vi "Process.vi"(8 "error in":errorcluster, 11 "Logger":refnum<class "Logger.PGSQL.lvclass">) -> (0 "error out":errorcluster, 3 "Logger out":refnum<class "Logger.PGSQL.lvclass">)   [LabVIEW 2019, in "Logger.PGSQL.lvlib" / "Logger.PGSQL.lvclass"]
doc: "---------------------------------------------------------------\nJKI State Machine Objects™\nhttp://jki.net/state-machine-objects/\nCopyright (C) 2005-2015, JKI <info@jki.net>\nALL RIGHTS RESERVED"
uses:
  Logger.PGSQL.lvclass
  <vilib>/JKI/JKI SMO/SMO/SMO.lvclass
  <userlib>/LevyLab/LV-Data/LV-Data.PG/LV-Data.PGSQL.lvclass
  <userlib>/LevyLab/LV-Data/LV-Data.PG/API/Write Variable (one-row).vi
  <userlib>/LevyLab/Logger/Logger/Logger.lvclass
  <userlib>/LevyLab/LV-Data/LV-Data.PG/API/Read Variable (string).vi
  C:/Program Files (x86)/National Instruments/LabVIEW 2019/user.lib/LevyLab/Logger/Logger/Logger.lvclass
  C:/Program Files (x86)/National Instruments/LabVIEW 2019/vi.lib/JKI/JKI SMO/SMO/SMO.lvclass
  <userlib>/LevyLab/Debug/Debug.lvlib
panel:
  out "State History":string
  out "Status":string
  out "Data":variant
  out "Address(es)":string
  # "DB Logger"
  # "For instructions on how to use the JKI State Machine Objects, examples and video tutorials, visit:\nhttp://jki.net/state-machine-objects/\n\nJKI State Machine Objects™\nhttp://jki.net/state-machine-objects/\nCopyright (C) 2005-2015, JKI <info@jki.net>\nALL RIGHTS RESERVED"
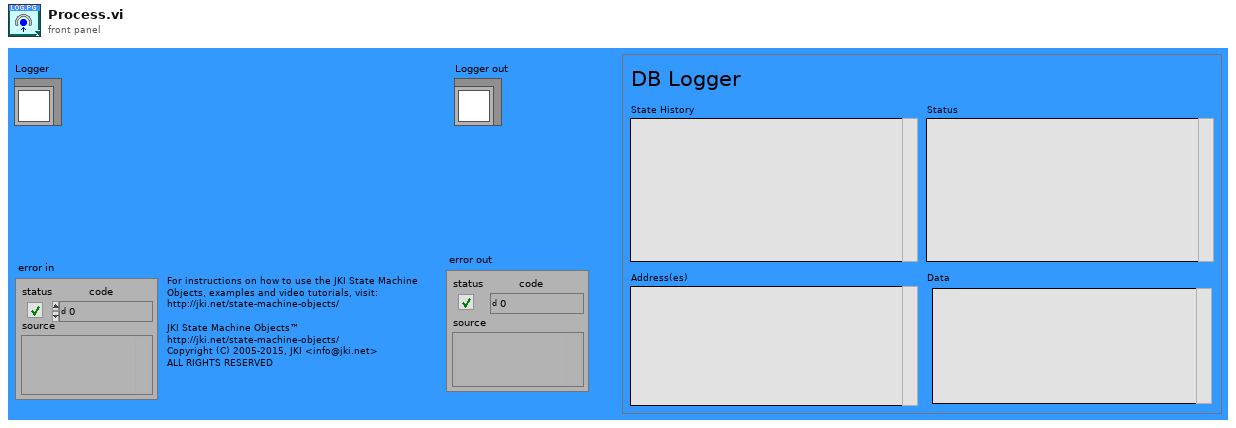
[diagram p1: front panel]
types:
  T1 = enum32{"invalid app kind", "Development System", "Run Time System", "Student Edition", "Embedded LabVIEW", "Evaluation", "Custom"}
  T2 = enum32{"Invalid", "Standard", "Closed", "Hidden", "Minimized", "Maximized"}
  T3 = cluster{"Core":cluster{"Current VI Reference":refnum<vi>, "Close Panel on Exit?":bool, "Last Error":cluster{"error":errorcluster, "previous state":string, "remaining states":string}, "Shutdown?":bool}, "SelfRef":refnum<class "Logger.PGSQL.lvclass">, "Data.PGSQL":refnum<class "LV-Data.PGSQL.lvclass">, "variable address":string, "data in":variant, "data out":variant, "Time":timestamp, "UI Behavior":string, "wait":u32}
  T4 = cluster{"Current VI Reference":refnum<vi>, "Close Panel on Exit?":bool, "Last Error":cluster{"error":errorcluster, "previous state":string, "remaining states":string}, "Shutdown?":bool}
  T5 = typedef "Debug.lvlib/Attribute.Debug.lvclass/DebugBehavior.ctl" = enum16{"Normal", "Debug"}
  T6 = typedef "smo.lvlib/SMO.lvclass/Protected Events.ctl" = cluster{"StopProcesses":refnum<user-event>, "AbortProcesses":refnum<user-event>, "Config Changed":refnum<user-event>, "Dependency":refnum<user-event>}
  T7 = typedef "Logger.PGSQL.lvlib/Logger.PGSQL.lvclass/PrivateEvents--Cluster.ctl" = cluster{"Set Address":refnum<user-event>, "Write Variable":refnum<user-event>, "Read Variable":refnum<user-event>}
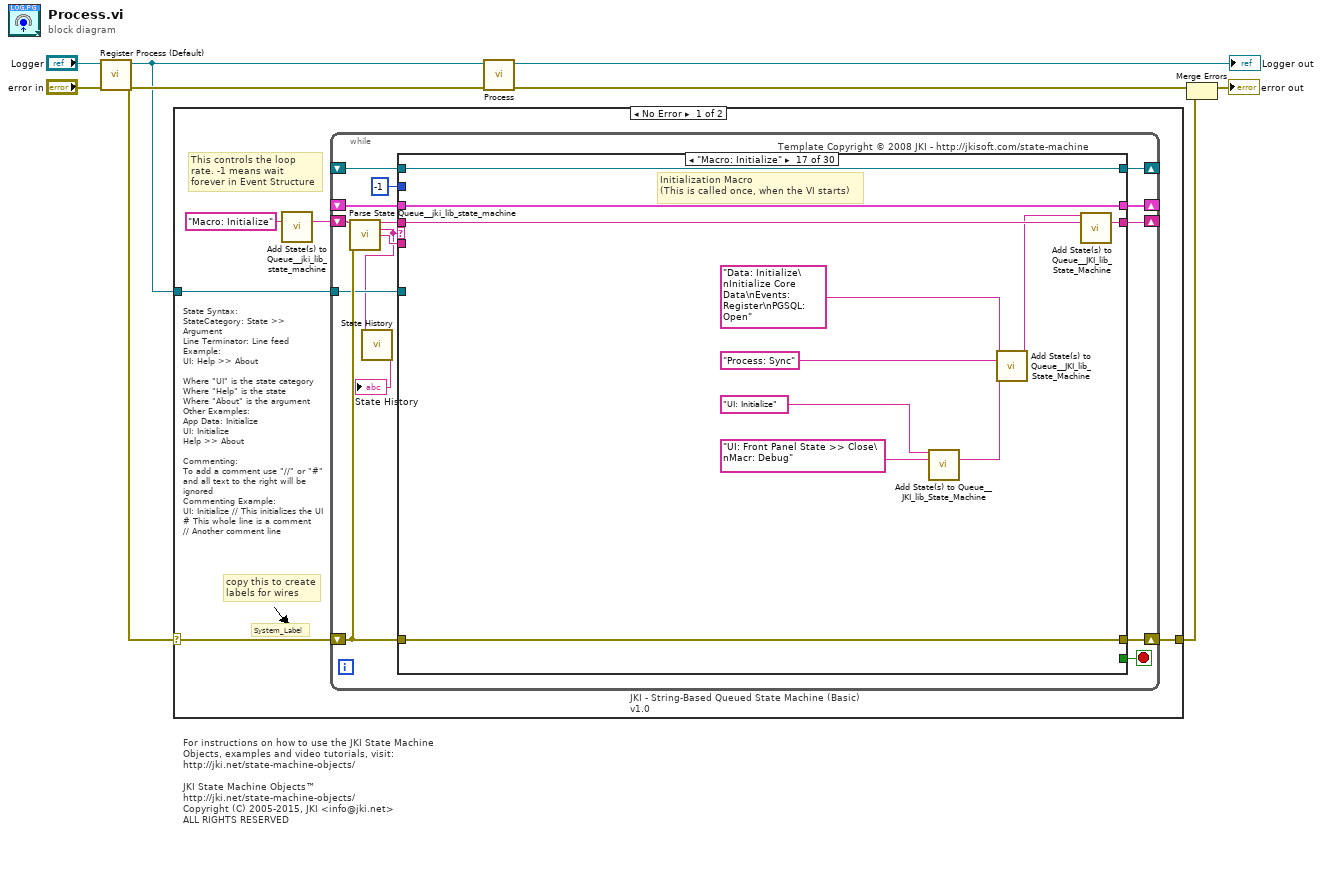
[diagram p0: block diagram]
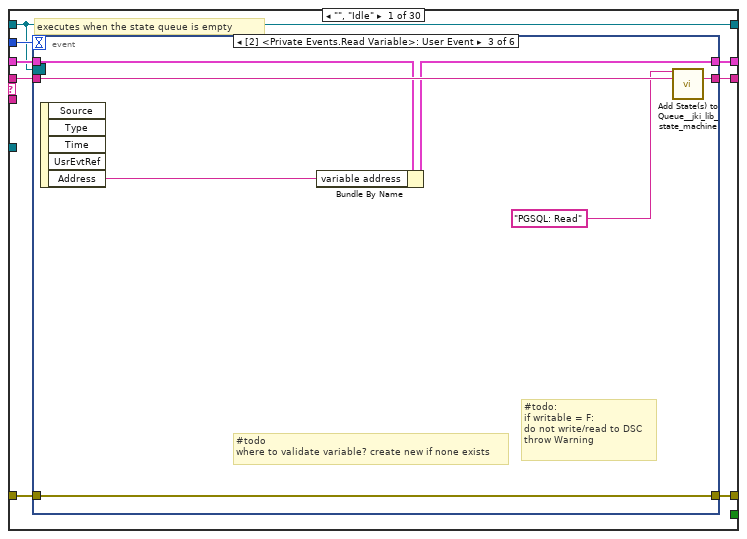
[diagram p2: hidden frame]
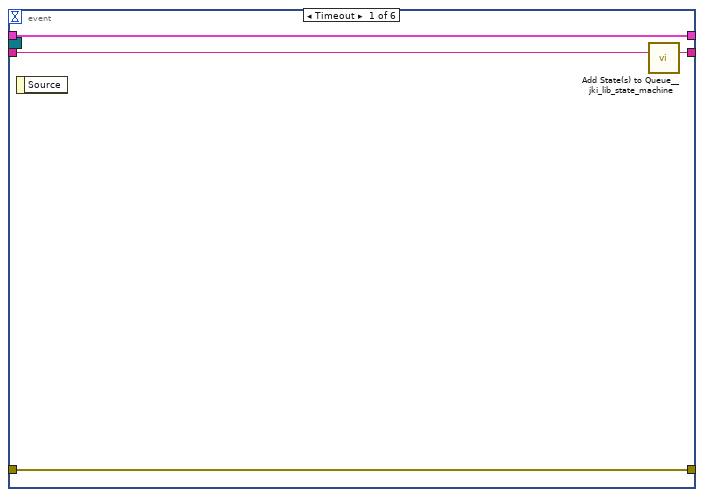
[diagram p3: hidden frame]
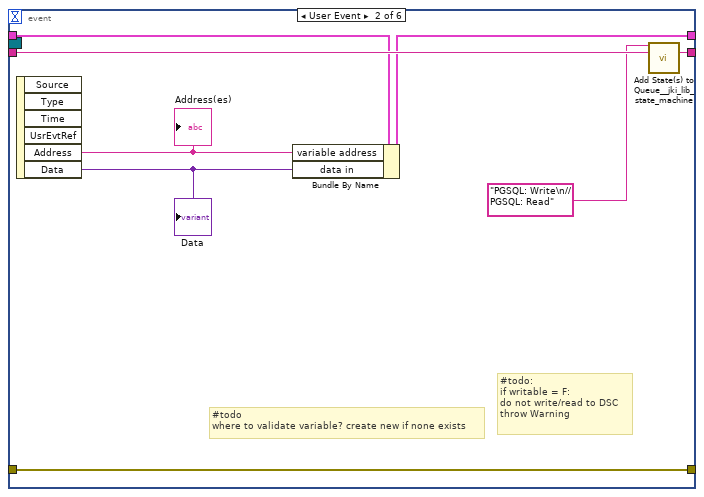
[diagram p4: hidden frame]
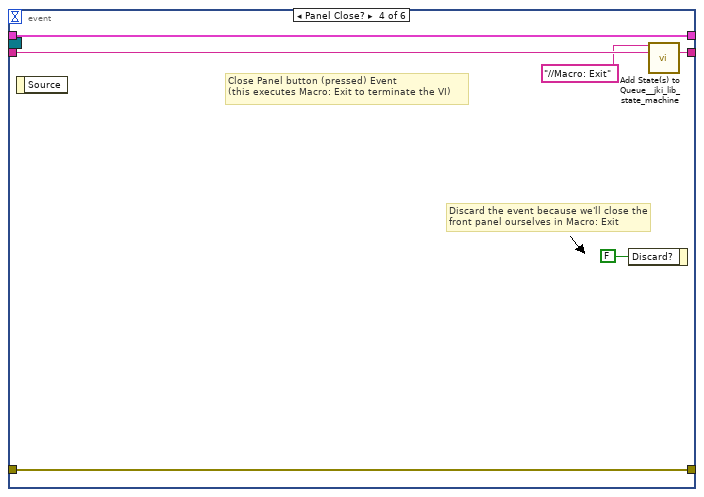
[diagram p5: hidden frame]
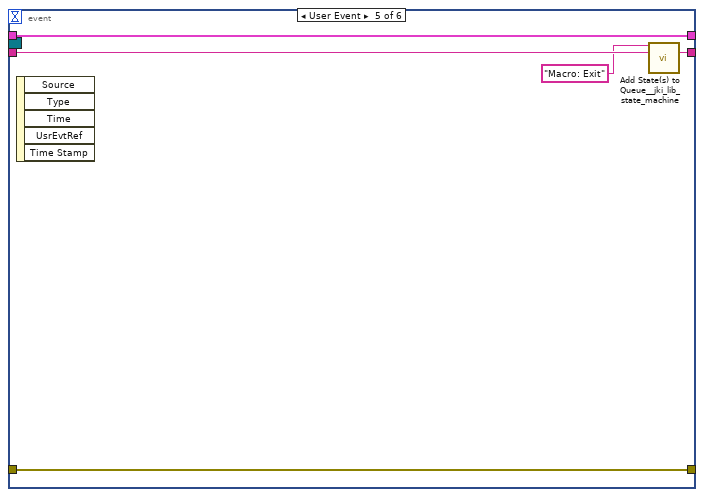
[diagram p6: hidden frame]
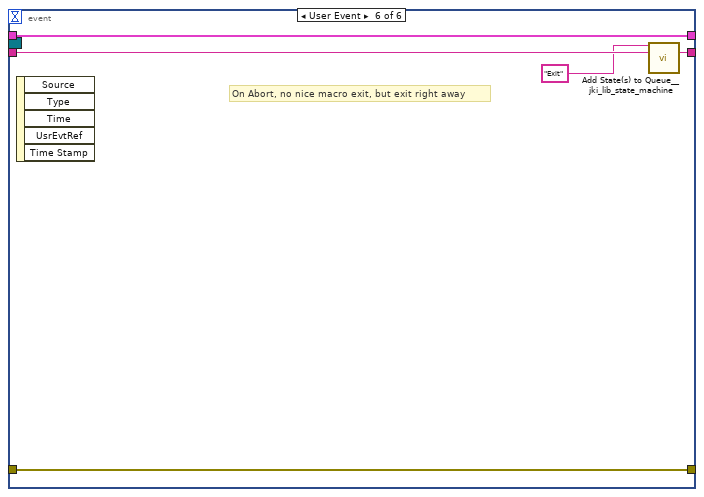
[diagram p7: hidden frame]
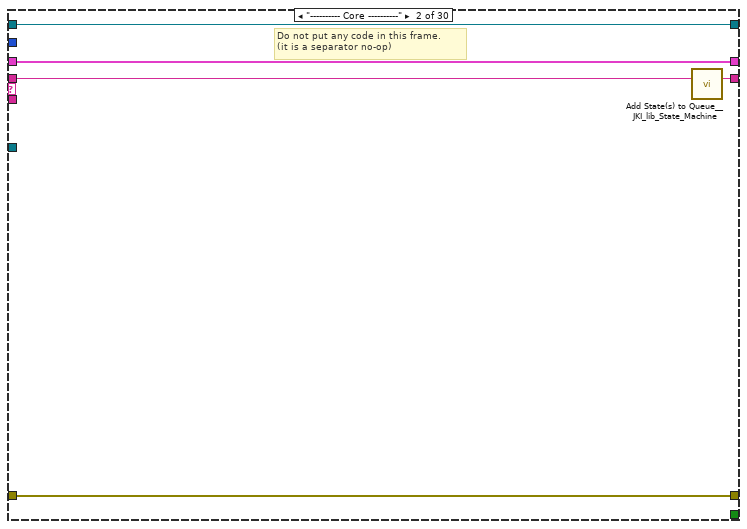
[diagram p8: hidden frame]
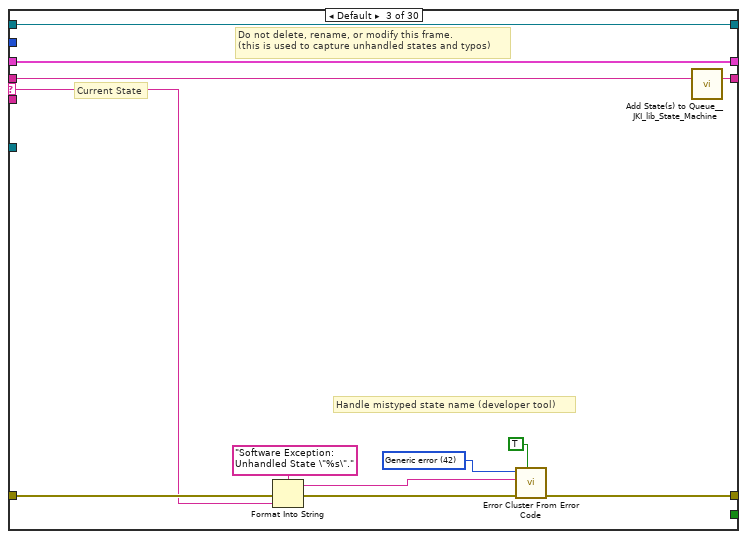
[diagram p9: hidden frame]
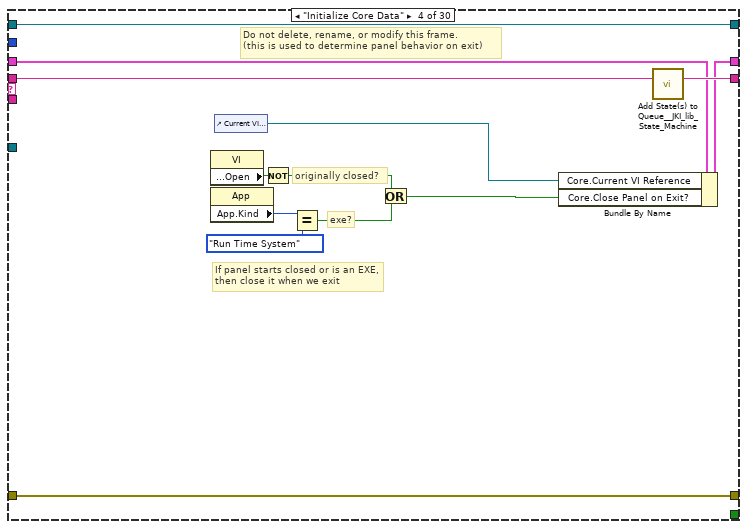
[diagram p10: hidden frame]
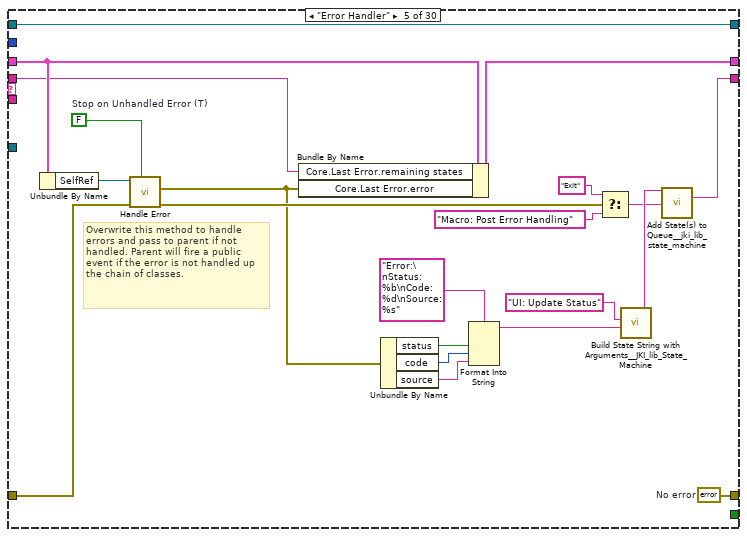
[diagram p11: hidden frame]
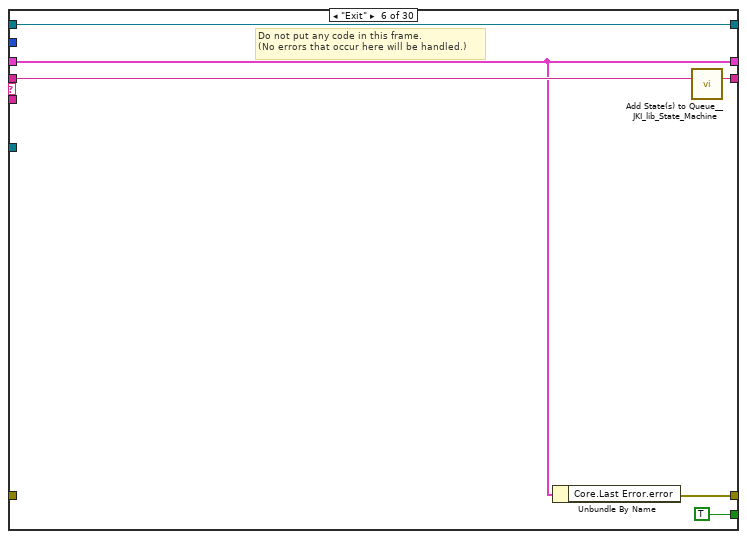
[diagram p12: hidden frame]
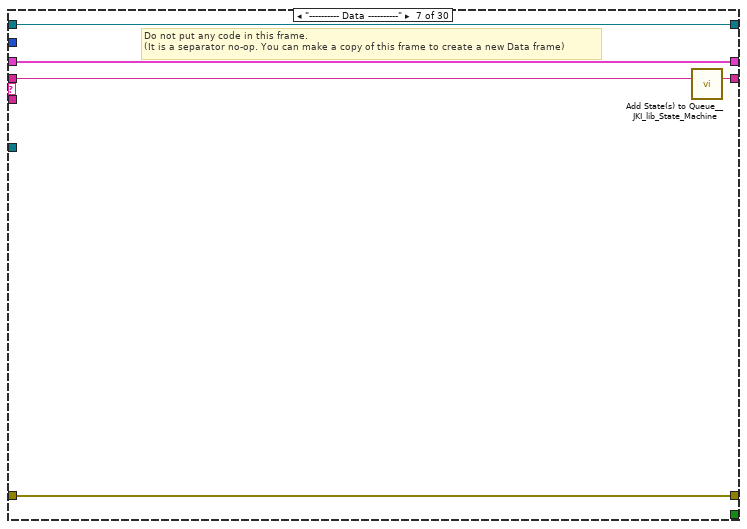
[diagram p13: hidden frame]
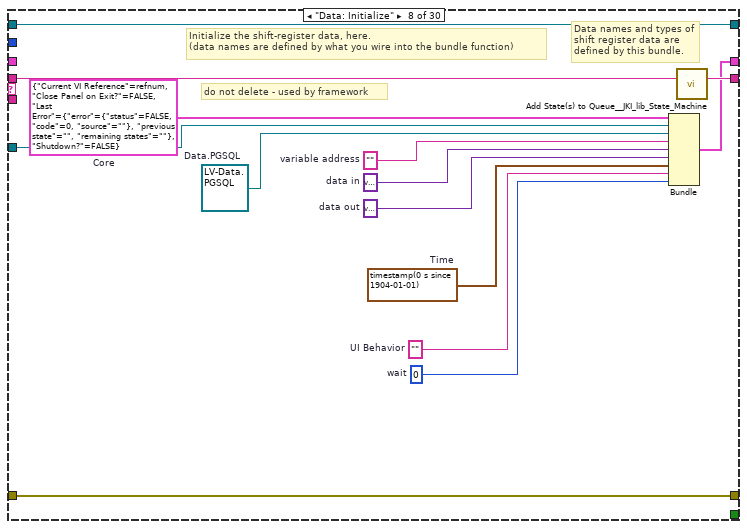
[diagram p14: hidden frame]
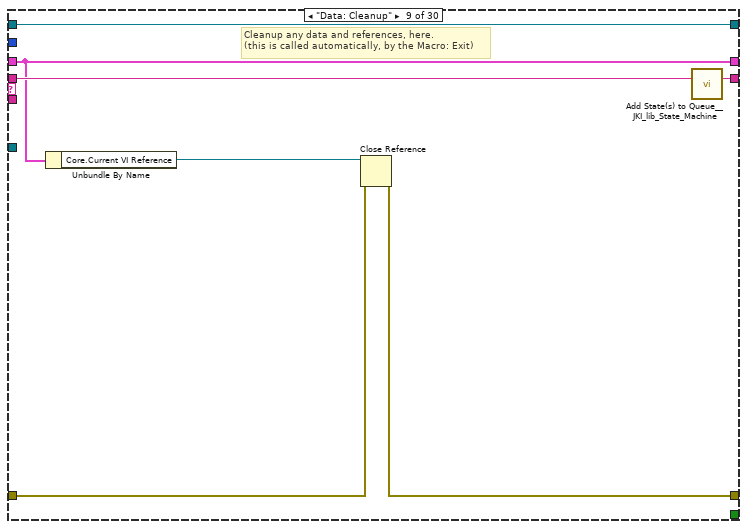
[diagram p15: hidden frame]
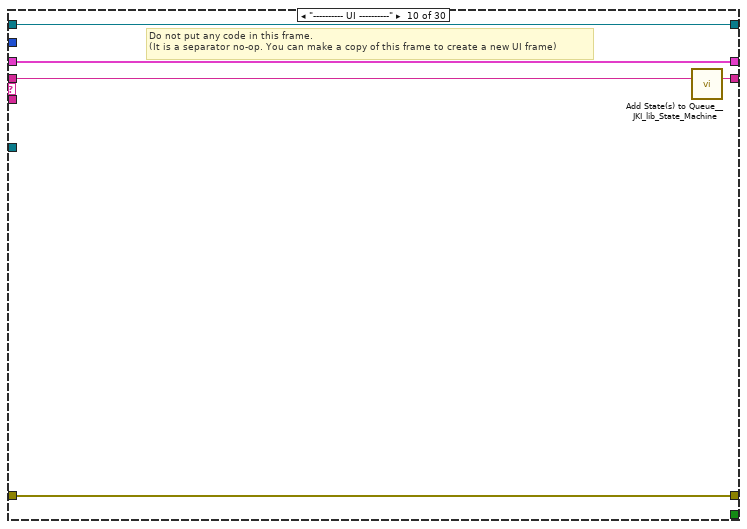
[diagram p16: hidden frame]
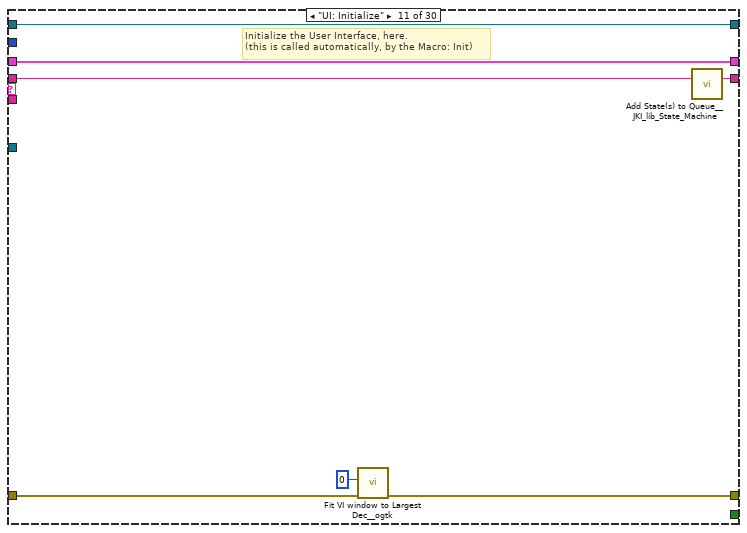
[diagram p17: hidden frame]
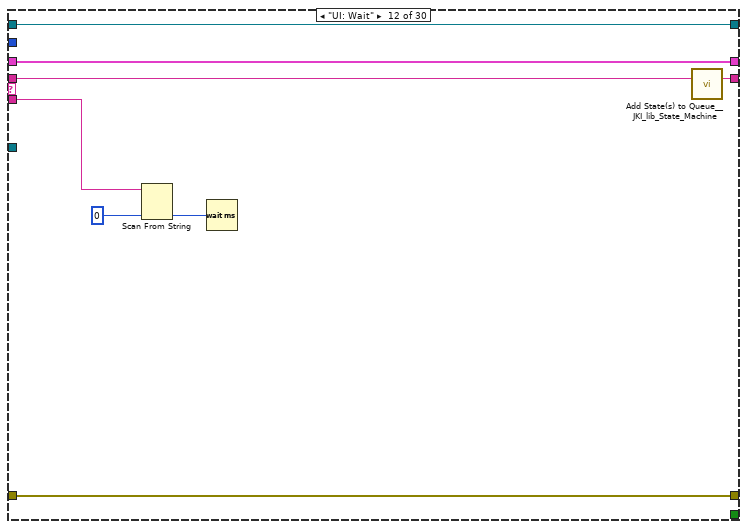
[diagram p18: hidden frame]
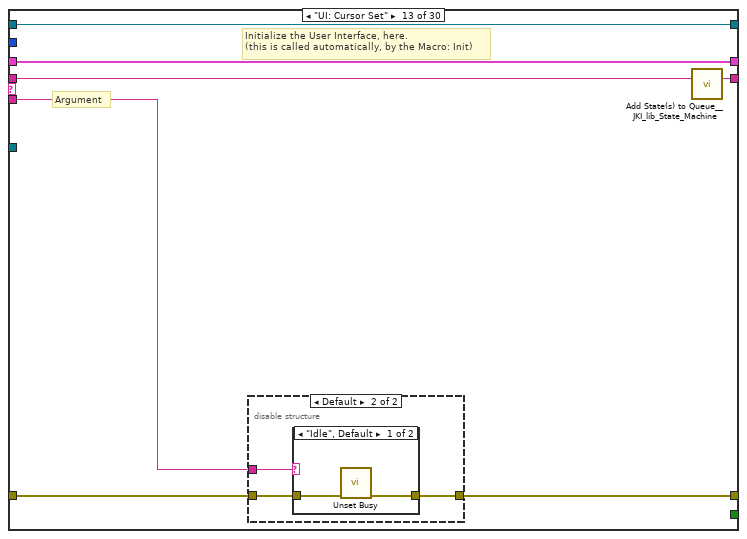
[diagram p19: hidden frame]
diagram:
  # "For instructions on how to use the JKI State Machine Objects, examples and video tutorials, visit:\nhttp://jki.net/state-machine-objects/\n\nJKI State Machine Objects™\nhttp://jki.net/state-machine-objects/\nCopyright (C) 2005-2015, JKI <info@jki.net>\nALL RIGHTS RESERVED"
  n1 = call <vilib>:"Register Process (Default).vi"("error in (no error)"="error in", "SMO"="Logger") -> ("error out"=w5:errorcluster, "SelfRef"=w4:refnum<class "Logger.PGSQL.lvclass">)  [unwired: 8 in]
  n2 = case shown="No Error" w5 {
    selector: w5 -> [w10 w424]
    tunnel: w4 -> [w11 _]
    tunnel: [w9 w424] -> w2
    frame No Error {
      # "State Syntax:\nStateCategory: State >> Argument\nLine Terminator: Line feed\nExample:\nUI: Help >> About\n\nWhere \"UI\" is the state category\nWhere \"Help\" is the state\nWhere \"About\" is the argument\nOther Examples:\nApp Data: Initialize\nUI: Initialize\nHelp >> About\n\nCommenting:\nTo add a comment use \"//\" or \"#\" and all text to the right will be ignored\nCommenting Example:\nUI: Initialize // This initializes the UI\n# This whole line is a comment\n// Another comment line"
      # "copy this to create labels for wires"
      # "This controls the loop rate. -1 means wait forever in Event Structure"
      # "System_Label"
      n3 = call <vilib>:"Add State(s) to Queue__jki_lib_state_machine.vi"("State(s) in (\"\")"="Macro: Initialize") -> ("States Out"=w13:string)  [unwired: 14 in]
      n4 = while "JKI - String-Based Queued State Machine (Basic) v1.0" {
        shift-right: [w22] -> _
        shift-left: _ -> [w21]
        shift-right: [w25] -> w9
        shift-left: w10 -> [w19]
        shift-right: [w24] -> _
        shift-left: w13 -> [w26]
        tunnel: w11 -> [w18]
        shift-right: [w17] -> _
        shift-left: _ -> [w16]
        stop <- w23 stop-if-true
        # "Template Copyright © 2008 JKI - http://jkisoft.com/state-machine"
        n5 = call <vilib>:"Parse State Queue__jki_lib_state_machine.vi"("State Queue"=w26, "Error In (no error)"=w19) -> ("Remaining States"=w28:string, "Current State"=w14:string, "Arguments"=w27:string)  [unwired: 11 in]
        n6 = call <userlib>:"State History.vi"("Current State"=w14) -> ("History"=→"State History":string)  [unwired: 10 in]
        n7 = case shown="\"Macro: Initialize\"" w14 {
          selector: w14 -> [_ _ w78 _ _ _ _ _ _ _ _ _ _ _ _ _ _ _ _ _ _ _ _ _ _ _ _ _ _ _]
          tunnel: w28 -> [w36 w76 w82 w101 w108 w128 w133 w147 w154 w159 w166 w174 w181 w196 w204 w236 w247 w261 w278 w298 w303 w314 w319 w332 w338 w343 w352 w376 w406 w423]
          tunnel: w27 -> [_ _ _ _ _ _ _ _ _ _ _ w168 w175 w190 w198 _ _ _ _ _ _ _ _ _ _ _ _ _ _ _]
          tunnel: w21 -> [w34 w73 w80 w92 w118 w124 w130 _ w149 w156 w164 w171 w179 w193 w200 w233 w241 w249 w268 w283 w300 w311 w316 w330 w336 w341 w344 w371 w399 w418]
          tunnel: [w33 w74 w84 w98 w119 w123 w131 w136 w150 w157 w162 w172 w176 w194 w201 w234 w237 w259 w276 w296 w301 w305 w317 w325 w334 w339 w347 w373 w403 w415] -> w25
          tunnel: w19 -> [w32 w74 w83 w98 w120 _ w131 w136 w151 w157 w161 w172 w177 w194 w202 w234 w237 w259 w276 w296 w301 w306 w317 w326 w334 w339 w345 w368 w400 w416]
          tunnel: [w35 w75 w81 w100 w104 w127 w132 w146 w153 w158 w165 w173 w180 w195 w203 w235 w246 w260 w277 w297 w302 w313 w318 w331 w337 w342 w351 w375 w405 w422] -> w24
          tunnel: [_ _ _ _ _ TRUE _ _ _ _ _ _ _ _ _ _ _ _ _ _ _ _ _ _ _ _ _ _ _ _] -> w23
          tunnel: [w31 w73 w80 w99 w117 w124 w130 w145 w149 w156 w164 w171 w179 w193 w200 w233 w241 w250 w269 w284 w300 w311 w316 w330 w336 w341 w349 w370 w399 w417] -> w22
          tunnel: -1 ("Timeout") -> [w30 _ _ _ _ _ _ _ _ _ _ _ _ _ _ _ _ _ _ _ _ _ _ _ _ _ _ _ _ _]
          tunnel: w18 -> [_ _ _ _ _ _ _ w137 _ _ _ _ _ _ _ _ _ _ _ _ _ _ _ _ _ _ _ _ _ _]
          tunnel: [w29 w72 w77 w89 w122 w125 w129 w144 w148 w155 w163 w170 w178 w192 w197 w232 w245 w258 w275 w291 w299 w312 w315 w329 w335 w340 w350 w374 w404 w421] -> w17
          tunnel: w16 -> [w29 w72 w77 w89 w122 w125 w129 w144 w148 w155 w163 w170 w178 w192 w197 w232 w245 w258 w275 w291 w299 w312 w315 _ w335 w340 w350 w374 w404 w421]
          frame "", "Idle" {
            # "executes when the state queue is empty"
            n8 = event shown="[2] <Private Events.Read Variable>: User Event" {
              selector: w29 -> [_ _ _ _ _ _]
              dyn-events: _ -> [_ _ _ _ _ _]
              timeout: w30 -> [_ _ _ _ _ _]
              tunnel: w36 -> [w40 w48 w55 w61 w66 w71]
              tunnel: [w39 w47 w54 w60 w65 w70] -> w35
              tunnel: w34 -> [w38 w45 w52 w58 w63 w68]
              tunnel: [w37 w46 w53 w59 w64 w69] -> w33
              tunnel: w32 -> [w37 w46 w53 w59 w64 w69]
              tunnel: [w38 w44 w51 w58 w63 w68] -> w31
              event Timeout {
                n9 = event-data() -> ()  [unwired: 1 in, 1 out]
                n10 = call <vilib>:"Add State(s) to Queue__jki_lib_state_machine.vi"("State(s) in (\"\")"=w40) -> ("States Out"=w39:string)  [unwired: 14 in]
              }
              event User Event {
                # "#todo:\nif writable = F:\ndo not write/read to DSC\nthrow Warning"
                # "#todo\nwhere to validate variable? create new if none exists"
                n11 = event-data() -> ("Address"=w41:string, "Data"=w42:variant)  [unwired: 1 in, 4 out]
                "Address(es)" <- w41
                "Data" <- w42
                n12 = Bundle By Name(cluster=w45, "variable address"=w41, "data in"=w42) -> (w44:T3)
                n13 = call <vilib>:"Add State(s) to Queue__jki_lib_state_machine.vi"("State(s) in Front (\"\")"="PGSQL: Write\n//PGSQL: Read" ("State(s) in Front (\"\")"), "State(s) in (\"\")"=w48) -> ("States Out"=w47:string)  [unwired: 13 in]
              }
              event User Event {
                # "#todo:\nif writable = F:\ndo not write/read to DSC\nthrow Warning"
                # "#todo\nwhere to validate variable? create new if none exists"
                n14 = event-data() -> ("Address"=w49:string)  [unwired: 1 in, 4 out]
                n15 = Bundle By Name(cluster=w52, "variable address"=w49) -> (w51:T3)
                n16 = call <vilib>:"Add State(s) to Queue__jki_lib_state_machine.vi"("State(s) in Front (\"\")"="PGSQL: Read" ("State(s) in Front (\"\")"), "State(s) in (\"\")"=w55) -> ("States Out"=w54:string)  [unwired: 13 in]
              }
              event Panel Close? {
                # "Discard the event because we'll close the front panel ourselves in Macro: Exit"
                # "Close Panel button (pressed) Event\n(this executes Macro: Exit to terminate the VI)"
                n17 = event-data() -> ()  [unwired: 1 in, 1 out]
                n18 = event-data("Discard?"=FALSE) -> ()  [unwired: 1 in, 1 out]
                n19 = call <vilib>:"Add State(s) to Queue__jki_lib_state_machine.vi"("State(s) in Front (\"\")"="//Macro: Exit", "State(s) in (\"\")"=w61) -> ("States Out"=w60:string)  [unwired: 13 in]
              }
              event User Event {
                n20 = event-data() -> ()  [unwired: 1 in, 5 out]
                n21 = call <vilib>:"Add State(s) to Queue__jki_lib_state_machine.vi"("State(s) in Front (\"\")"="Macro: Exit", "State(s) in (\"\")"=w66) -> ("States Out"=w65:string)  [unwired: 13 in]
              }
              event User Event {
                # "On Abort, no nice macro exit, but exit right away"
                n22 = event-data() -> ()  [unwired: 1 in, 5 out]
                n23 = call <vilib>:"Add State(s) to Queue__jki_lib_state_machine.vi"("State(s) in Front (\"\")"="Exit", "State(s) in (\"\")"=w71) -> ("States Out"=w70:string)  [unwired: 13 in]
              }
            }
          }
          frame "---------- Core ----------" {
            # "Do not put any code in this frame.\n(it is a separator no-op)"
            n24 = call <vilib>:"Add State(s) to Queue__JKI_lib_State_Machine.vi"("State(s) in (\"\")"=w76) -> ("States Out"=w75:string)  [unwired: 14 in]
          }
          frame Default {
            w87 = 42 items=["No error", "Argument error", "Memory is full", "Out of zone", "End of file", "File already open", "Generic file I/O error", "File not found", "File permission error", "Disk is full", "Duplicate path", "Too many files open", "System feature not enabled", "Resource file not found", "Cannot add resource", "Resource not found", "Image not found", "Image memory error", "Pen does not exist", "Config type invalid", "Config token not found", "Config parse error", "Config memory error", "Bad external code format", "Bad external code offset", "External code not present", "Null window", "Destroy window error", "Null menu", "Print aborted", "Bad print record", "Print driver error", "Windows error during printing", "Memory error during printing", "Print dialog error", "Generic print error", "Invalid device refnum", "Device not found", "Device parameter error", "Device unit error", "Cannot open device", "Device call aborted", "Generic error", "Cancelled by user", "Object ID too low", "Object ID too high", "Object not in heap", "Unknown heap", "Unknown object (invalid DefProc)", "Unknown object (DefProc not in table)", "Message out of range", "Invalid (null) method", "Unknown message", "Manager call not supported", "Bad address", "Network operation in progress", "Network operation timed out", "Connection is busy", "Network attribute not supported", "Network error", "Address in use", "System out of memory", "Connection aborted", "Connection refused", "Not connected", "Already connected", "Connection closed", "Initialization error (interapplication manager)", "Bad occurrence", "Wait on unbound occurrence handler", "Occurrence queue overflow", "Datalog type conflict", "Unused", "Unrecognized type (interapplication manager)", "Memory corrupt", "Failed to make temporary DLL", "Old CIN version", "Drag socket not found", "Failed to load drop-object", "Failed to register OLE object", "Failed to release OLE object", "Format specifier type mismatch", "Unknown format specifier", "Too few format specifiers", "Too many format specifiers", "Scan failed", "Newer CIN version", "Error converting to variant", "Runtime menu error", "Password tampered", "Variant attribute not found", "Incompatible variant data type", "Event data is not available", "Event Store is not present", "Occurrence is not found", "Event Queue is not created", "Event info is not available", "Refnum passed is NULL", "Error retrieving Class GUID", "Error retrieving CoClass GUID", "Error retrieving TypeLib GUID.", "Bad built application magic bytes.", "Specific driver is different from the specific driver associated with the Logical Name.", "There is no session opened to the class driver.", "Max Error", "MAX - Error with config objects", "MAX - Error loading configuration", "MAX - Group not supported"]
            # "Current State"
            # "Do not delete, rename, or modify this frame.\n(this is used to capture unhandled states and typos)"
            # "Handle mistyped state name (developer tool)"
            n25 = Format Into String(format string="Software Exception: Unhandled State \"%s\"." ("message"), error in=w83, w78) -> (resulting string=w86:string, error out=w85:errorcluster)  [unwired: 1 in]
            n26 = call <vilib>:"Error Cluster From Error Code.vi"("show call chain? (False)"=TRUE, "error in (no error)"=w85, "error message (\"\")"=w86, "error code (0)"=w87) -> ("error out"=w84:errorcluster)  [unwired: 5 in]
            n27 = call <vilib>:"Add State(s) to Queue__JKI_lib_State_Machine.vi"("State(s) in (\"\")"=w82) -> ("States Out"=w81:string)  [unwired: 14 in]
          }
          frame "Initialize Core Data" {
            # "Do not delete, rename, or modify this frame.\n(this is used to determine panel behavior on exit)"
            # "originally closed?"
            # "exe?"
            # "If panel starts closed or is an EXE, then close it when we exit"
            n28 = property class="VI"() -> ("Front Panel.Open"=w97:bool)  [unwired: 2 in, 2 out]
            n29 = property class="App"() -> ("App.Kind"=w96:T1)  [unwired: 2 in, 2 out]
            n30 = control-ref of="Current VI Reference"() -> (w90:refnum<vi>)
            n31 = Not(x=w97) -> (.not. x?=w94:bool)
            n32 = Equal?(x=w96, y=T1."Run Time System" ("Application:Kind")) -> (x = y?=w93:bool)
            n33 = Or(x=w94, y=w93) -> (x .or. y?=w91:bool)
            n34 = Bundle By Name(cluster=w92, "Core.Current VI Reference"=w90, "Core.Close Panel on Exit?"=w91) -> (w99:T3)
            n35 = call <vilib>:"Add State(s) to Queue__JKI_lib_State_Machine.vi"("State(s) in (\"\")"=w101) -> ("States Out"=w100:string)  [unwired: 14 in]
          }
          frame "Error Handler" {
            w114 = FALSE  # Stop on Unhandled Error (T)
            w119 = errorcluster {"status"=FALSE, "code"=0, "source"=""}  # No error
            # "Overwrite this method to handle errors and pass to parent if not handled. Parent will fire a public event if the error is not handled up the chain of classes."
            n36 = Unbundle By Name(w118) -> ("SelfRef"=w121:refnum<class "Logger.PGSQL.lvclass">)
            n37 = call-dynamic "Handle Error.vi"("Stop on Unhandled Error (T)"=w114, "error in"=w120, "SMO"=w121) -> ("handling error"=w115:errorcluster, "Unhandled error"=w113:errorcluster)  [unwired: 6 in, 1 out]
            n38 = Bundle By Name(cluster=w118, "Core.Last Error.remaining states"=w108, "Core.Last Error.error"=w113) -> (w117:T3)
            n39 = Unbundle By Name(w113) -> ("status"=w112:bool, "code"=w110:i32, "source"=w109:string)
            n40 = Format Into String(format string="Error:\nStatus: %b\nCode: %d\nSource: %s", w112, w110, w109) -> (resulting string=w103:string)  [unwired: 2 in, 1 out]
            n41 = Select(t="Exit", s=w115, f="Macro: Post Error Handling") -> (s? t:f=w105:string)
            n42 = call <vilib>:"Build State String with Arguments__JKI_lib_State_Machine.vi"("Arguments (\"\")"=w103, "State"="UI: Update Status") -> ("State with Arguments"=w106:string)  [unwired: 4 in]
            n43 = call <vilib>:"Add State(s) to Queue__jki_lib_state_machine.vi"("State(s) in Front (\"\")"=w106, "State(s) at Back (\"\")"=w105) -> ("States Out"=w104:string)  [unwired: 13 in]
          }
          frame "Exit" {
            # "Do not put any code in this frame.\n(No errors that occur here will be handled.)"
            n44 = Unbundle By Name(w124) -> ("Core.Last Error.error"=w123:errorcluster)
            n45 = call <vilib>:"Add State(s) to Queue__JKI_lib_State_Machine.vi"("State(s) in (\"\")"=w128) -> ("States Out"=w127:string)  [unwired: 14 in]
          }
          frame "---------- Data ----------" {
            # "Do not put any code in this frame.\n(It is a separator no-op. You can make a copy of this frame to create a new Data frame)"
            n46 = call <vilib>:"Add State(s) to Queue__JKI_lib_State_Machine.vi"("State(s) in (\"\")"=w133) -> ("States Out"=w132:string)  [unwired: 14 in]
          }
          frame "Data: Initialize" {
            w134 = u32 0  # wait
            w135 = ""  # UI Behavior
            w138 = timestamp(0 s since 1904-01-01)  # Time
            w139 = refnum<class "LV-Data.PGSQL.lvclass"> refnum  # Data.PGSQL
            w140 = variant  # data out
            w141 = variant  # data in
            w142 = ""  # variable address
            w143 = T4 {"Current VI Reference"=refnum, "Close Panel on Exit?"=FALSE, "Last Error"={"error"={"status"=FALSE, "code"=0, "source"=""}, "previous state"="", "remaining states"=""}, "Shutdown?"=FALSE}  # Core
            # "do not delete - used by framework"
            # "Data names and types of shift register data are defined by this bundle."
            # "Initialize the shift-register data, here.\n(data names are defined by what you wire into the bundle function)"
            n47 = Bundle("Core"=w143, "SelfRef"=w137, "Data.PGSQL"=w139, "variable address"=w142, "data in"=w141, "data out"=w140, "Time"=w138, "UI Behavior"=w135, "wait"=w134) -> (w145:T3)  [unwired: 1 in]
            n48 = call <vilib>:"Add State(s) to Queue__JKI_lib_State_Machine.vi"("State(s) in (\"\")"=w147) -> ("States Out"=w146:string)  [unwired: 14 in]
          }
          frame "Data: Cleanup" {
            # "Cleanup any data and references, here.\n(this is called automatically, by the Macro: Exit)"
            n49 = Unbundle By Name(w149) -> ("Core.Current VI Reference"=w152:refnum<vi>)
            n50 = Close Reference(reference=w152, error in (no error)=w151) -> (error out=w150:errorcluster)
            n51 = call <vilib>:"Add State(s) to Queue__JKI_lib_State_Machine.vi"("State(s) in (\"\")"=w154) -> ("States Out"=w153:string)  [unwired: 14 in]
          }
          frame "---------- UI ----------" {
            # "Do not put any code in this frame.\n(It is a separator no-op. You can make a copy of this frame to create a new UI frame)"
            n52 = call <vilib>:"Add State(s) to Queue__JKI_lib_State_Machine.vi"("State(s) in (\"\")"=w159) -> ("States Out"=w158:string)  [unwired: 14 in]
          }
          frame "UI: Initialize" {
            # "Initialize the User Interface, here.\n(this is called automatically, by the Macro: Init)"
            n53 = call <userlib>:"Fit VI window to Largest Dec__ogtk.vi"("error in (no error)"=w161, "border spacing (2 px)"=0) -> ("error out"=w162:errorcluster)  [unwired: 4 in, 1 out]
            n54 = call <vilib>:"Add State(s) to Queue__JKI_lib_State_Machine.vi"("State(s) in (\"\")"=w166) -> ("States Out"=w165:string)  [unwired: 14 in]
          }
          frame "UI: Wait" {
            n55 = Scan From String(input string=w168, default 1=u32 0) -> (output 1=w167:u32)  [unwired: 3 in, 3 out]
            n56 = Wait (ms)(milliseconds to wait=w167) -> ()  [unwired: 1 out]
            n57 = call <vilib>:"Add State(s) to Queue__JKI_lib_State_Machine.vi"("State(s) in (\"\")"=w174) -> ("States Out"=w173:string)  [unwired: 14 in]
          }
          frame "UI: Cursor Set" {
            # "Argument"
            # "Initialize the User Interface, here.\n(this is called automatically, by the Macro: Init)"
            n58 = disable-structure shown="Default" {
              disable-tunnel: w177 -> [w182 w185]
              disable-tunnel: [w182 w184] -> w176
              disable-tunnel: w175 -> [_ w183]
              frame condition #0 {
              }
              frame condition #1 (active) {
                n59 = case shown="\"Idle\", Default" w183 {
                  tunnel: w185 -> [w187 w189]
                  tunnel: [w186 w188] -> w184
                  frame "Idle", Default {
                    n60 = call <vilib>:"Unset Busy.vi"("error in (no error)"=w187) -> ("error out"=w186:errorcluster)  [unwired: 10 in]
                  }
                  frame "Busy" {
                    n61 = call <vilib>:"Set Busy.vi"("error in (no error)"=w189) -> ("error out"=w188:errorcluster)  [unwired: 9 in, 1 out]
                  }
                }
              }
            }
            n62 = call <vilib>:"Add State(s) to Queue__JKI_lib_State_Machine.vi"("State(s) in (\"\")"=w181) -> ("States Out"=w180:string)  [unwired: 14 in]
          }
          frame "UI: Update Status" {
            # "Do not put any code in this frame.\n(It is a separator no-op. You can make a copy of this frame to create a new UI frame)"
            n63 = call <userlib>:"State History.vi"("Current State"=w190) -> ("History"=→"Status":string)  [unwired: 10 in]
            n64 = call <vilib>:"Add State(s) to Queue__JKI_lib_State_Machine.vi"("State(s) in (\"\")"=w196) -> ("States Out"=w195:string)  [unwired: 14 in]
          }
          frame "UI: Front Panel State" {
            # "Argument"
            # "Set Front Panel Open or Closed\n(Usage: \"UI: Front Panel State >> Open|Close\")"
            n65 = Unbundle By Name(w200) -> ("Core.Current VI Reference"=w199:refnum<vi>)
            n66 = disable-structure shown="Default" {
              disable-tunnel: w202 -> [w208 w231]
              disable-tunnel: [w207 w231] -> w201
              disable-tunnel: w199 -> [w206 _]
              disable-tunnel: w198 -> [w205 _]
              frame condition #0 (active) {
                n67 = case shown="\"Close\"" w205 {
                  tunnel: w208 -> [w212 w225]
                  tunnel: [w214 w226] -> w207
                  tunnel: w206 -> [w213 w223]
                  frame "Open", Default {
                    n68 = property class="VI"(reference=w213, error in=w212) -> (reference out=w210:refnum<vi>, error out=w211:errorcluster, "FP.State"=w209:T2)
                    n69 = case shown="\"Closed\"" w209 {
                      tunnel: [w217 w220] -> w214
                      tunnel: w211 -> [w216 w220]
                      tunnel: w210 -> [w215 _]
                      frame "Closed" {
                        n70 = invoke class="VI" method="FP.Open"(reference=w215, error in=w216, "Activate"=TRUE, "State"=T2."Standard") -> (error out=w217:errorcluster)  [unwired: 1 in, 4 out]
                      }
                      frame Default {
                      }
                    }
                  }
                  frame "Close" {
                    n71 = property class="VI"(reference=w223, error in=w225) -> (reference out=w222:refnum<vi>, error out=w224:errorcluster, "FP.State"=w221:T2)
                    n72 = case shown="Default" w221 {
                      tunnel: [w227 w230] -> w226
                      tunnel: w224 -> [w227 w229]
                      tunnel: w222 -> [_ w228]
                      frame "Invalid", "Closed" {
                      }
                      frame Default {
                        n73 = invoke class="VI" method="FP.Close"(reference=w228, error in=w229) -> (error out=w230:errorcluster)  [unwired: 1 in, 2 out]
                      }
                    }
                  }
                }
              }
              frame condition #1 {
              }
            }
            n74 = call <vilib>:"Add State(s) to Queue__JKI_lib_State_Machine.vi"("State(s) in (\"\")"=w204) -> ("States Out"=w203:string)  [unwired: 14 in]
          }
          frame "---------- Macro ----------" {
            # "Do not put any code in this frame.\n(It is a separator no-op. You can make a copy of this frame to create a new Macro frame)"
            n75 = call <vilib>:"Add State(s) to Queue__JKI_lib_State_Machine.vi"("State(s) in (\"\")"=w236) -> ("States Out"=w235:string)  [unwired: 14 in]
          }
          frame "Macro: Initialize" {
            # "Initialization Macro\n(This is called once, when the VI starts)"
            n76 = call <vilib>:"Add State(s) to Queue__JKI_lib_State_Machine.vi"("State(s) in Front (\"\")"="UI: Initialize", "State(s) in (\"\")"="UI: Front Panel State >> Close\nMacr: Debug") -> ("States Out"=w239:string)  [unwired: 13 in]
            n77 = call <vilib>:"Add State(s) to Queue__JKI_lib_State_Machine.vi"("State(s) in Front (\"\")"="Data: Initialize\nInitialize Core Data\nEvents: Register\nPGSQL: Open", "State(s) in (\"\")"="Process: Sync", "State(s) at Back (\"\")"=w239) -> ("States Out"=w243:string)  [unwired: 12 in]
            n78 = call <vilib>:"Add State(s) to Queue__JKI_lib_State_Machine.vi"("State(s) in Front (\"\")"=w243, "State(s) in (\"\")"=w247) -> ("States Out"=w246:string)  [unwired: 13 in]
          }
          frame "Macro: Debug" {
            # "exe?"
            # "If pane is an EXE, then close it when we exit"
            # "Macro: Debug\n(get debug behavior, determine UI and determine shutdown behavior)"
            n79 = Unbundle By Name(w249) -> ("Core.Close Panel on Exit?"=w252:bool, "SelfRef"=w257:refnum<class "Logger.PGSQL.lvclass">)
            n80 = property class="App"() -> ("App.Kind"=w255:T1)  [unwired: 2 in, 2 out]
            n81 = Equal?(x=w255, y=T1."Run Time System" ("Application:Kind")) -> (x = y?=w251:bool)
            n82 = call <userlib>:"Get Debug Mode.vi"("SMO"=w257) -> ("Behavior"=w256:T5)  [unwired: 8 in, 2 out]
            n83 = case shown="\"Debug\"" w256 {
              tunnel: [_ "UI: Front Panel State >> Open\nUI: Wait >> 1000"] -> w248
              tunnel: [w262 w263] -> w253
              tunnel: w252 -> [w262 _]
              tunnel: w251 -> [_ w265]
              frame "Normal", Default {
                # "respect core.close"
              }
              frame "Debug" {
                # "keep panel open\nunless exe"
                n84 = Or(x=w265, y=FALSE) -> (x .or. y?=w263:bool)
              }
            }
            n85 = Bundle By Name(cluster=w249, "Core.Close Panel on Exit?"=w253) -> (w250:T3)
            n86 = call <vilib>:"Add State(s) to Queue__JKI_lib_State_Machine.vi"("State(s) in Front (\"\")"=w248, "State(s) in (\"\")"=w261) -> ("States Out"=w260:string)  [unwired: 13 in]
          }
          frame "Macro: Post Error Handling" {
            # "Clear Last Error?"
            n87 = Unbundle By Name(w268) -> ("Core.Last Error.remaining states"=w270:string, "Core.Shutdown?"=w271:bool)
            n88 = Unbundle By Name(w268) -> ("Core.Last Error.error"=w274:errorcluster)
            n89 = case shown="False" FALSE {
              tunnel: w274 -> [w282 _]
              tunnel: [w282 _] -> w273
              frame False {
              }
              frame True {
              }
            }
            n90 = case shown="True" w271 {
              tunnel: w270 -> [w279 w281]
              tunnel: [w279 w280] -> w267
              frame False {
                # "These are the remaining states (at the moment the error occured). States can be altered according to business logic."
                # "NOT SHUTTING DOWN"
              }
              frame True {
                # "Developer can decide to alter the states but should be aware that during the shutdown process, there are certain states that must be run for the SMO to properly shut itself (and this process) down. As such, one can add states to perform additional clean-ups, but should append the remaining state to be executed."
                # "SHUTTING DOWN"
                n91 = call <vilib>:"Add State(s) to Queue__jki_lib_state_machine.vi"("State(s) in (\"\")"=w281) -> ("States Out"=w280:string)  [unwired: 14 in]
              }
            }
            n92 = Bundle By Name(cluster=w268, "Core.Last Error.error"=w273) -> (w269:T3)
            n93 = call <vilib>:"Add State(s) to Queue__JKI_lib_State_Machine.vi"("State(s) in Front (\"\")"=w267, "State(s) in (\"\")"=w278) -> ("States Out"=w277:string)  [unwired: 13 in]
          }
          frame "Macro: Exit" {
            # "Exit Macro\n(This is called once, when the VI exits)"
            n94 = Unbundle By Name(w283) -> ("Core.Close Panel on Exit?"=w295:bool)
            n95 = Bundle By Name(cluster=w283, "Core.Shutdown?"=TRUE) -> (w284:T3)
            n96 = Select(t="UI: Front Panel State >> Close", s=w295, f="") -> (s? t:f=w293:string)
            n97 = call <vilib>:"Add State(s) to Queue__JKI_lib_State_Machine.vi"("State(s) in Front (\"\")"="PGSQL: Close\nData: Cleanup\nEvents: Unregister", "State(s) in (\"\")"="Process: Sync", "State(s) at Back (\"\")"="Exit") -> ("States Out"=w288:string)  [unwired: 12 in]
            n98 = call <vilib>:"Add State(s) to Queue__JKI_lib_State_Machine.vi"("State(s) in (\"\")"=w293, "State(s) at Back (\"\")"=w288) -> ("States Out"=w292:string)  [unwired: 13 in]
            n99 = call <vilib>:"Add State(s) to Queue__JKI_lib_State_Machine.vi"("State(s) in Front (\"\")"=w292, "State(s) in (\"\")"=w298) -> ("States Out"=w297:string)  [unwired: 13 in]
          }
          frame "---------- Process ----------" {
            # "Template Separator\n(You can make a copy of, or modify, this frame)"
            n100 = call <vilib>:"Add State(s) to Queue__JKI_lib_State_Machine.vi"("State(s) in (\"\")"=w303) -> ("States Out"=w302:string)  [unwired: 14 in]
          }
          frame "Process: Sync" {
            n101 = Unbundle By Name(w311) -> ("SelfRef"=w307:refnum<class "Logger.PGSQL.lvclass">)
            n102 = call <vilib>:"WaitOnProcessSync.vi"("error in (no error)"=w306, "SMO"=w307) -> ("error out"=w305:errorcluster, "Don't run?"=w310:bool)  [unwired: 7 in, 1 out]
            n103 = Select(t="Data: Cleanup\nEvents: Unregister\nExit", s=w310, f="") -> (s? t:f=w304:string)
            n104 = call <vilib>:"Add State(s) to Queue__JKI_lib_State_Machine.vi"("State(s) in Front (\"\")"=w304, "State(s) in (\"\")"=w314) -> ("States Out"=w313:string)  [unwired: 13 in]
          }
          frame "---------- Events ----------" {
            # "Template Separator\n(You can make a copy of, or modify, this frame)"
            n105 = call <vilib>:"Add State(s) to Queue__JKI_lib_State_Machine.vi"("State(s) in (\"\")"=w319) -> ("States Out"=w318:string)  [unwired: 14 in]
          }
          frame "Events: Register" {
            # "Expand to add\nmore events"
            n106 = Unbundle By Name(w330) -> ("SelfRef"=w327:refnum<class "Logger.PGSQL.lvclass">)
            n107 = call <vilib>:"GetProtectedEvents.vi"("SMO"=w327) -> ("error out"=w323:errorcluster, "SMO Protected Events"=w328:T6, "SMO"=w322:refnum<class "Logger.PGSQL.lvclass">)  [unwired: 8 in]
            n108 = call "Logger.GetPrivateEvents.vi"("Logger"=w322) -> ("error out"=w320:errorcluster, "Private Events"=w321:T7)  [unwired: 8 in, 1 out]
            n109 = register-events(w328, w321) -> (reference out=w329:refnum<event-registration>, error out=w324:errorcluster)  [unwired: 2 in]
            n110 = Merge Errors(w320, w326, w324, w323) -> (w325:errorcluster)
            n111 = call <vilib>:"Add State(s) to Queue__JKI_lib_State_Machine.vi"("State(s) in (\"\")"=w332) -> ("States Out"=w331:string)  [unwired: 14 in]
          }
          frame "Events: Unregister" {
            n112 = Unregister For Events(event registration refnum=w335, error in=w334) -> (error out=w333:errorcluster)
            n113 = call <vilib>:"Clear Errors.vi"("error in (no error)"=w333) -> ()  [unwired: 5 in, 2 out]
            n114 = call <vilib>:"Add State(s) to Queue__JKI_lib_State_Machine.vi"("State(s) in (\"\")"=w338) -> ("States Out"=w337:string)  [unwired: 14 in]
          }
          frame "---------- PGSQL ----------" {
            n115 = call <vilib>:"Add State(s) to Queue__JKI_lib_State_Machine.vi"("State(s) in (\"\")"=w343) -> ("States Out"=w342:string)  [unwired: 14 in]
          }
          frame "PGSQL: Open" {
            n116 = Unbundle By Name(w344) -> ("Data.PGSQL"=w346:refnum<class "LV-Data.PGSQL.lvclass">)
            n117 = call <userlib>:"PGSQL.Open.vi"("error in (no error)"=w345, "Data.PG in"=w346) -> ("error out"=w347:errorcluster, "Data.PG out"=w348:refnum<class "LV-Data.PGSQL.lvclass">)  [unwired: 8 in]
            n118 = Bundle By Name(cluster=w344, "Data.PGSQL"=w348) -> (w349:T3)
            n119 = call <vilib>:"Add State(s) to Queue__JKI_lib_State_Machine.vi"("State(s) in (\"\")"=w352) -> ("States Out"=w351:string)  [unwired: 14 in]
          }
          frame "PGSQL: Write" {
            n120 = Unbundle By Name(w371) -> ("Data.PGSQL"=w367:refnum<class "LV-Data.PGSQL.lvclass">, "variable address"=w366:string, "data in"=w365:variant, "Time"=w361:timestamp)
            n121 = call "Write Or Not.vi"("Time"=w361, "data in"=w365) -> ("Write?"=w363:bool)  [unwired: 1 in]
            n122 = case shown="True" w363 {
              tunnel: [w379 w390] -> w373
              tunnel: [w382 w397] -> w372
              tunnel: w368 -> [w379 w396]
              tunnel: w367 -> [w382 w395]
              tunnel: w366 -> [_ w394]
              tunnel: [TRUE ("Wrote to DB?") w385] -> w362
              tunnel: w365 -> [_ w392]
              tunnel: [w381 w389] -> w364
              tunnel: w361 -> [w381 _]
              tunnel: ["Write Not Attempted" w384] -> w360
              tunnel: [w377 w383] -> w358
              frame False {
                n123 = Get Date/Time In Seconds() -> (seconds since 1Jan1904=w377:timestamp)
              }
              frame True {
                n124 = call "Shorten Cluster.vi"("error in (no error)"=w396, "Variant"=w392, "variable address in"=w394) -> ("error out"=w391:errorcluster, "Variant"=w388:variant, "variable address out"=w393:string)
                n125 = Get Date/Time In Seconds() -> (seconds since 1Jan1904=w389:timestamp)
                n126 = call-poly <userlib>:"Write Variable.vi"("error in (no error)"=w391, "Data"=w388, "variable"=w393, "Data.PG in"=w395) -> ("error out"=w390:errorcluster, "Wrote to DB?"=w385:bool, "Data.PG out"=w397:refnum<class "LV-Data.PGSQL.lvclass">)  [unwired: 4 in, 1 out]
                n127 = Select(t="Write Succesful", s=w385, f="Write Failed") -> (s? t:f=w384:string)
                n128 = Get Date/Time In Seconds() -> (seconds since 1Jan1904=w383:timestamp)
              }
            }
            n129 = Format Into String(w360, w358) -> (resulting string=w357:string)  [unwired: 3 in, 1 out]
            n130 = Bundle By Name(cluster=w371, "Data.PGSQL"=w372, "Time"=w364) -> (w370:T3)
            n131 = call <vilib>:"Build State String with Arguments__JKI_lib_State_Machine.vi"("Arguments (\"\")"=w357, "State"="UI: Update Status") -> ("State with Arguments"=w353:string)  [unwired: 4 in]
            n132 = Select(t="", s=w362, f="PGSQL: Close\nPGSQL: Open") -> (s? t:f=w356:string)
            n133 = call <vilib>:"Add State(s) to Queue__jki_lib_state_machine.vi"("State(s) in Front (\"\")"=w353, "State(s) at Back (\"\")"=w356) -> ("States Out"=w354:string)  [unwired: 13 in]
            n134 = call <vilib>:"Add State(s) to Queue__JKI_lib_State_Machine.vi"("State(s) in Front (\"\")"=w354, "State(s) in (\"\")"=w376) -> ("States Out"=w375:string)  [unwired: 13 in]
          }
          frame "PGSQL: Read" {
            n135 = Unbundle By Name(w399) -> ("SelfRef"=w402:refnum<class "Logger.PGSQL.lvclass">, "Data.PGSQL"=w401:refnum<class "LV-Data.PGSQL.lvclass">, "variable address"=w398:string)
            n136 = case shown="Default" w398 {
              selector: w398 -> [_ w408]
              tunnel: [w407 w414] -> w403
              tunnel: w402 -> [_ w413]
              tunnel: w401 -> [_ w410]
              tunnel: w400 -> [w407 w409]
              frame "" {
              }
              frame Default {
                n137 = call-poly <userlib>:"Read Variable.vi"("error in (no error)"=w409, "PG path"=w408, "Data.PGQL in"=w410) -> ("error out"=w411:errorcluster, "Value"=w412:string)  [unwired: 3 in, 4 out]
                n138 = call "Logger.ReadVariable.vi"("error in (no error)"=w411, "Data"=w412, "Address"=w408, "Logger"=w413) -> ("error out"=w414:errorcluster)  [unwired: 6 in, 1 out]
              }
            }
            n139 = call <vilib>:"Add State(s) to Queue__JKI_lib_State_Machine.vi"("State(s) in (\"\")"=w406) -> ("States Out"=w405:string)  [unwired: 14 in]
          }
          frame "PGSQL: Close" {
            n140 = Unbundle By Name(w418) -> ("Data.PGSQL"=w420:refnum<class "LV-Data.PGSQL.lvclass">)
            n141 = call-dynamic "Close.vi"("error in (no error)"=w416, "Data.PG in"=w420) -> ("error out"=w415:errorcluster, "Data.PG out"=w419:refnum<class "LV-Data.PGSQL.lvclass">)  [unwired: 8 in]
            n142 = Bundle By Name(cluster=w418, "Data.PGSQL"=w419) -> (w417:T3)
            n143 = call <vilib>:"Add State(s) to Queue__JKI_lib_State_Machine.vi"("State(s) in (\"\")"=w423) -> ("States Out"=w422:string)  [unwired: 14 in]
          }
        }
      }
    }
    frame Error {
    }
  }
  n144 = call-parent "Process.vi"("error in"=w5, "Logger"=w4) -> ("error out"=w3:errorcluster, "Logger out"=→"Logger out":refnum<class "Logger.PGSQL.lvclass">)  [unwired: 8 in]
  n145 = Merge Errors(w3, w2) -> (→"error out":errorcluster)
